vi "HDI Fiducial.vi"(5 "error in (no error)":errorcluster, 6 "Image Src":T1) -> (0 "Matched?":bool, 1 "y rel move":dbl, 2 "x rel move":dbl, 3 "Score":dbl, 4 "error out":errorcluster)   [LabVIEW 2011]
uses:
  <vilib>/vision/Pattern Matching.llb/IMAQ GM Match Report.ctl
  <vilib>/vision/Image Controls.llb/IMAQ Image.ctl
  <vilib>/vision/Pattern Matching.llb/IMAQ Curve Parameters.ctl
  <vilib>/vision/Pattern Matching.llb/IMAQ Match Range Setting.ctl
  <vilib>/vision/NI_Vision_Development_Module.lvlib
panel:
  in  "Scale Factor":sgl=0.000429
  out "y":sgl
  out "x":sgl
  out "Image Out":T1(plugin-control)
  out "Calibrated Matches (Geometric Matching 1)":T2[](array[typedef]) {"Correlation Score" format="%.2f"; "Target Template Curve Score" format="%.2f"; "Template Target Curve Score" format="%.2f"; "Bounding Box"."y" format="%.2f"; "Bounding Box"."x" format="%.2f"; "Position"."y" format="%.2f"; "Position"."x" format="%.2f"; "Score" format="%.2f"; "Scale" format="%.2f"; "Angle" format="%.2f"; "Occlusion %" format="%.2f"}
  out "Matches (Geometric Matching 1)":T2[](array[typedef]) {"Correlation Score" format="%.2f"; "Target Template Curve Score" format="%.2f"; "Template Target Curve Score" format="%.2f"; "Bounding Box"."y" format="%.2f"; "Bounding Box"."x" format="%.2f"; "Position"."y" format="%.2f"; "Position"."x" format="%.2f"; "Score" format="%.2f"; "Scale" format="%.2f"; "Angle" format="%.2f"; "Occlusion %" format="%.2f"}
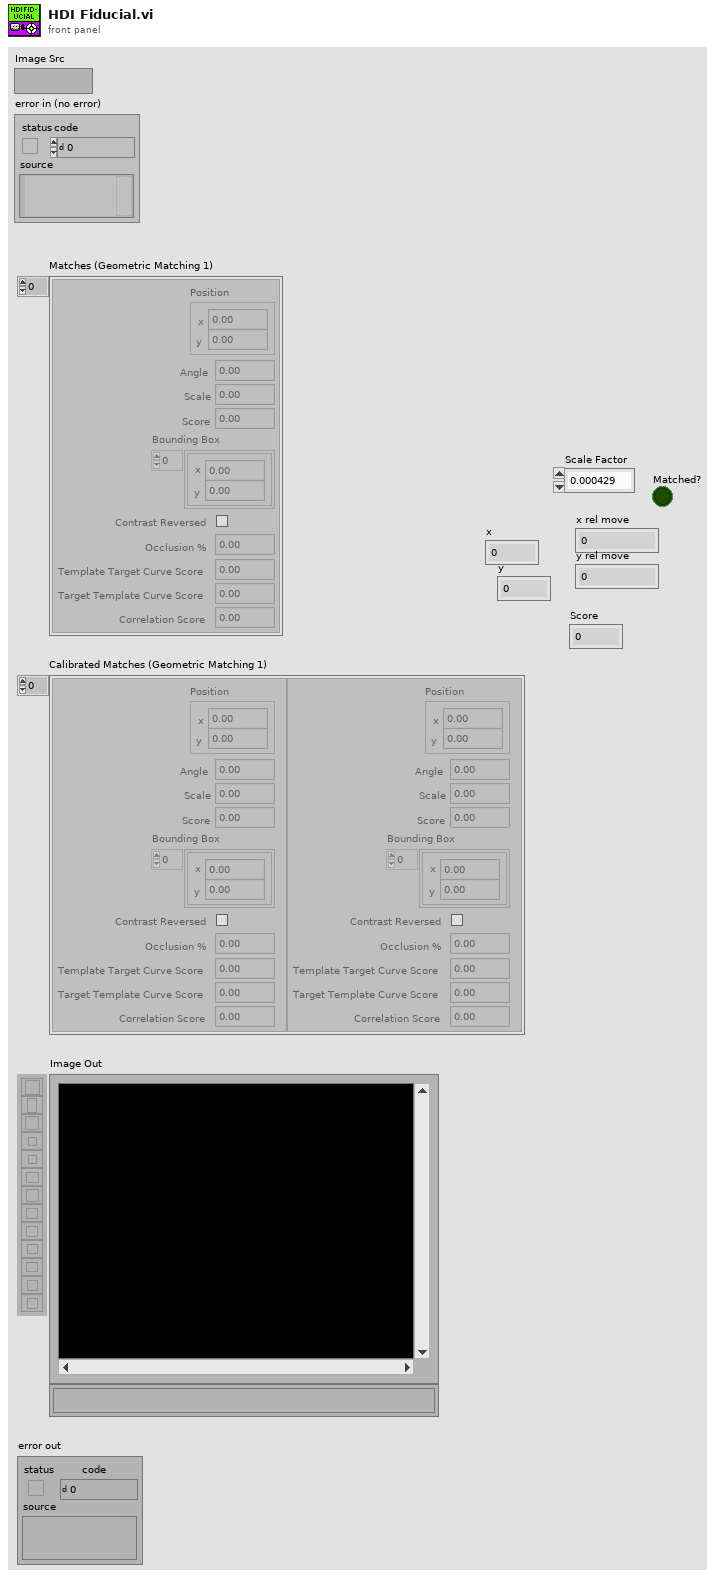
[diagram p1: front panel]
types:
  T1 = typedef "IMAQ Image.ctl" = refnum<image>
  T2 = typedef "IMAQ GM Match Report.ctl" = cluster{"Position":cluster{"x":sgl, "y":sgl}, "Angle":sgl, "Scale":sgl, "Score":sgl, "Bounding Box":cluster{"x":sgl, "y":sgl}[], "Contrast Reversed":bool, "Occlusion %":sgl, "Template Target Curve Score":sgl, "Target Template Curve Score":sgl, "Correlation Score":sgl}
  T3 = typedef "IMAQ Curve Parameters.ctl" = cluster{"Extraction Mode":u32, "Edge Threshold":i32, "Edge Filter Size":u32, "Min Length":i32, "Row Search Step Size":i32, "Col Search Step Size":i32, "Max Endpoint Gap":i32, "Closed":bool, "Subpixel":bool}
  T4 = typedef "IMAQ Match Range Setting.ctl" = cluster{"Match Constraints":u32, "Min":dbl, "Max":dbl}
  T5 = cluster{"Curve Parameters":T3, "Match Mode":cluster{"Rotation":bool, "Scale":bool, "Occlusion":bool, "Reserved":bool, "Reserved":bool, "Reserved":bool}, "Range Settings":T4[], "Number of Matches":i32, "Minimum Match Score":sgl, "SubPixel Accuracy":bool, "Adv. Geometric Match Options 2":cluster{"Setup Data Item":u16, "Item Value":dbl}[]}
  T6 = cluster{"Global Rectangle":i32[], "Contours":cluster{"ID":enum32{"External", "Internal"}, "Type":u32, "Coordinates":i32[]}[]}
  T7 = cluster{"histogram":u32[], "Minimal Value":sgl, "Maximal Value":sgl, "Starting Value":sgl, "Interval Width":sgl, "Mean Value":sgl, "Standard  Variation":sgl, "Area (pixels)":i32}
  T8 = typedef "Image Type" = u32
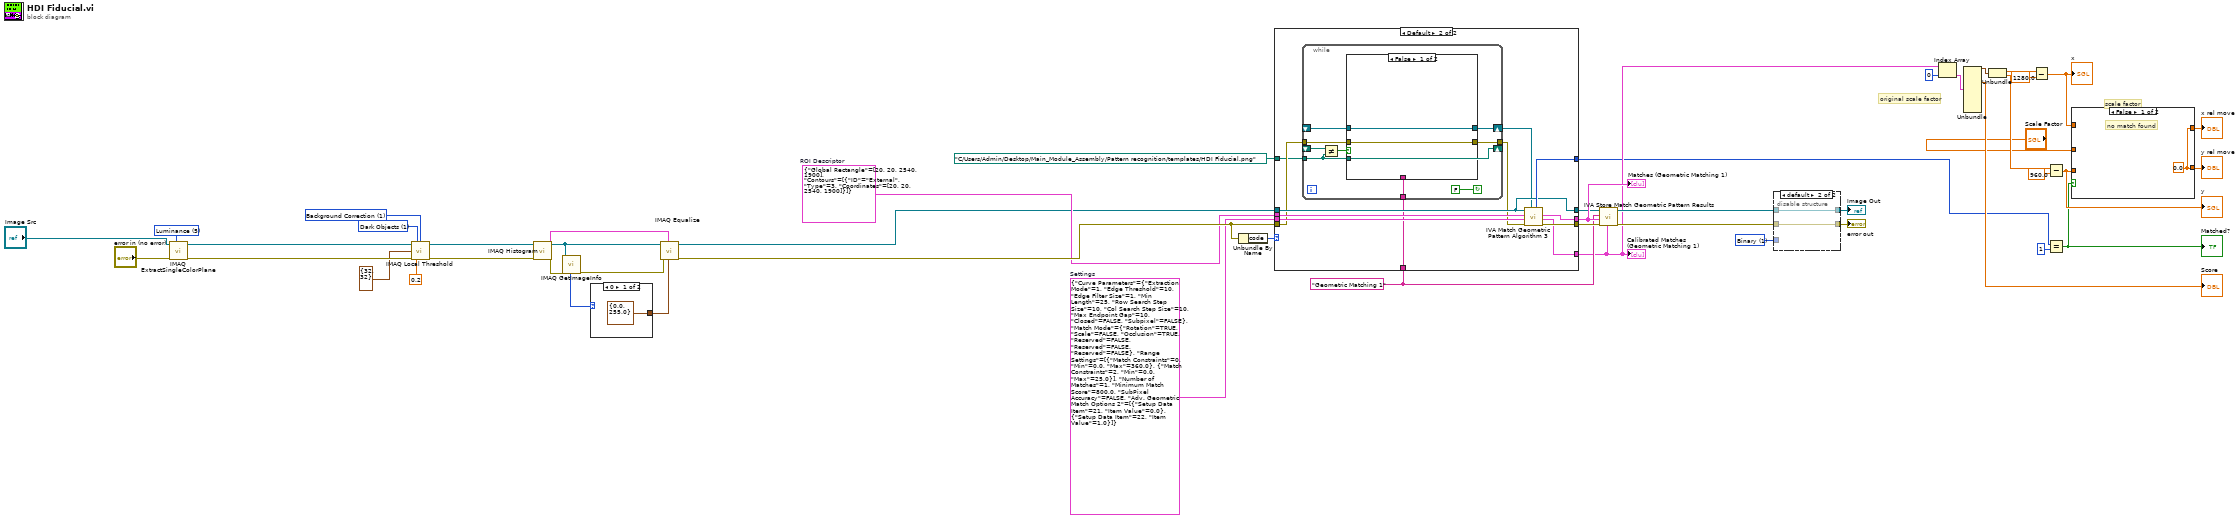
[diagram p0: block diagram]
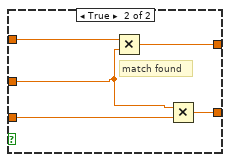
[diagram p2: hidden frame]
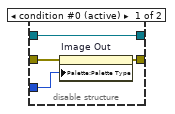
[diagram p3: hidden frame]
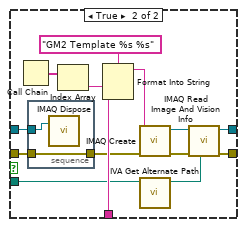
[diagram p5: hidden frame]
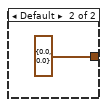
[diagram p6: hidden frame]
diagram:
  w20 = u32 1 items=["Grayscale", "Binary", "Gradient", "Rainbow", "Temperature", "User Defined"] ("Palette")
  w25 = T5 {"Curve Parameters"={"Extraction Mode"=1, "Edge Threshold"=10, "Edge Filter Size"=1, "Min Length"=25, "Row Search Step Size"=10, "Col Search Step Size"=10, "Max Endpoint Gap"=10, "Closed"=FALSE, "Subpixel"=FALSE}, "Match Mode"={"Rotation"=TRUE, "Scale"=FALSE, "Occlusion"=TRUE, "Reserved"=FALSE, "Reserved"=FALSE, "Reserved"=FALSE}, "Range Settings"=[{"Match Constraints"=0, "Min"=0.0, "Max"=360.0}, {"Match Constraints"=2, "Min"=0.0, "Max"=25.0}], "Number of Matches"=1, "Minimum Match Score"=800.0, "SubPixel Accuracy"=FALSE, "Adv. Geometric Match Options 2"=[{"Setup Data Item"=21, "Item Value"=0.0}, {"Setup Data Item"=22, "Item Value"=1.0}]}  # Settings
  w24 = "Geometric Matching 1" ("Step Name")
  w32 = T6 {"Global Rectangle"=[20, 20, 2540, 1900], "Contours"=[{"ID"=enum."External", "Type"=3, "Coordinates"=[20, 20, 2540, 1900]}]}  # ROI Descriptor
  w42 = u32 1 items=["Bright Objects", "Dark Objects"] ("Look For (Bright Objects)")
  w45 = u32 1 items=["Niblack", "Background Correction"] ("Method")
  w48 = 5 items=["Red", "Green", "Blue", "Hue", "Saturation", "Luminance", "Value", "Intensity"] ("Color Plane")
  # "original scale factor"
  # "scale factor"
  n1 = call "IMAQ ExtractSingleColorPlane"("Color Plane"=w48, "error in (no error)"="error in (no error)", "Image Src"="Image Src") -> ("error out"=w47:errorcluster, "Image Dst Out"=w46:T1)  [unwired: 1 in, 6 out]
  n2 = call "IMAQ Local Threshold"("Image Src"=w46, "Look For (Bright Objects)"=w42, "Method (Niblack)"=w45, "Window Size (32x32)"=cluster{"SizeX":i32, "SizeY":i32} {"SizeX"=32, "SizeY"=32} ("Kernel Size"), "error in (no error)"=w47, "Niblack Deviation Factor (0.2)"=0.2 ("Niblack Deviation Factor")) -> ("Image Dst Out"=w37:T1, "error out"=w41:errorcluster)  [unwired: 2 in, 6 out]
  n3 = call "IMAQ Histogram"("error in (no error)"=w41, "Image"=w37) -> ("error out"=w36:errorcluster, "Histogram Report"=w39:T7)  [unwired: 3 in, 5 out]
  n4 = call "IMAQ GetImageInfo"("error in (no error)"=w36, "Image"=w37) -> ("error out"=w35:errorcluster, "Image Type"=w38:T8)  [unwired: 8 out]
  n5 = case shown="0" w38 {
    tunnel: [cluster{"Minimum":sgl, "Maximum":sgl} {"Minimum"=0.0, "Maximum"=255.0} ("Range") cluster{"Minimum":sgl, "Maximum":sgl} {"Minimum"=0.0, "Maximum"=0.0} ("Range")] -> w34
    frame 0 {
    }
    frame Default {
    }
  }
  n6 = call "IMAQ Equalize"("Range"=w34, "Histogram Report"=w39, "error in (no error)"=w35, "Image Src"=w37) -> ("error out"=w40:errorcluster, "Image Dst Out"=w31:T1)  [unwired: 2 in, 4 out]
  n7 = Unbundle By Name(w40) -> ("code"=w27:i32)
  n8 = case shown="Default" w27 {
    tunnel: path "C:/Users/Admin/Desktop/Main_Module_Assembly/Pattern recognition/templates/HDI Fiducial.png" ("Template File Path") -> [_ w53]
    tunnel: w40 -> [_ w54]
    tunnel: w25 -> [_ w63]
    tunnel: w32 -> [_ w62]
    tunnel: w31 -> [w51 w57]
    tunnel: [_ w61] -> w30
    tunnel: [_ w60] -> w28
    tunnel: [_ w59] -> w4
    tunnel: [_ w58] -> w3
    tunnel: [w51 w57] -> w26
    tunnel: w24 -> [_ w52]
    frame -1074396199, -1074396198 {
      # "Discard Coordinate System Error"
    }
    frame Default {
      n9 = while {
        shift-right: [w72] -> w55
        shift-left: _ -> [w71]
        tunnel: [w69] -> w56
        tunnel: w54 -> [w68]
        tunnel: w53 -> [w64]
        tunnel: w52 -> [w67]
        shift-right: [w64] -> _
        shift-left: _ -> [w66]
        stop <- FALSE continue-if-true
        n10 = Not Equal?(x=w66, y=w64) -> (x != y?=w65:bool)
        n11 = case shown="False" w65 {
          tunnel: [w74 w86] -> w72
          tunnel: w71 -> [w74 w78]
          tunnel: [w73 w83] -> w69
          tunnel: w68 -> [w73 w79]
          tunnel: w67 -> [_ w80]
          tunnel: w64 -> [_ w76]
          frame False {
          }
          frame True {
            n12 = Call Chain() -> (call chain=w82:string[])
            n13 = stacked-sequence {
              tunnel: w79 -> [w90]
              tunnel: w78 -> [w89]
              tunnel: [w90] -> w77
              frame #0 {
                n14 = call "IMAQ Dispose"("Image"=w89) -> ()  [unwired: 2 in, 4 out]
              }
            }
            n15 = Index Array(array=w82) -> (element=w81:string)  [unwired: 1 in]
            n16 = Format Into String(format string="GM2 Template %s %s" ("Image Name"), w81, w80) -> (resulting string=w88:string)  [unwired: 2 in, 1 out]
            n17 = call "IMAQ Create"("Image Name"=w88, "error in (no error)"=w77) -> ("New Image"=w85:T1, "error out"=w84:errorcluster)  [unwired: 2 in, 1 out]
            n18 = call <vilib>:"IVA Get Alternate Path.vi"("Path In"=w76) -> ("Path Out"=w75:path)  [unwired: 10 out]
            n19 = call "IMAQ Read Image And Vision Info"("File Path"=w75, "error in (no error)"=w84, "Image"=w85) -> ("error out"=w83:errorcluster, "Image Out"=w86:T1)  [unwired: 1 in, 6 out]
          }
        }
      }
      n20 = call <vilib>:"IVA Match Geometric Pattern Algorithm 3.vi"("Template"=w55, "error in (no error)"=w56, "Settings"=w63, "ROI Descriptor"=w62, "Image"=w57) -> ("error out"=w61:errorcluster, "Calibrated Matches"=w59:T2[], "Matches"=w60:T2[], "Number of Matches"=w58:i32)  [unwired: 3 out]
    }
  }
  "Matches (Geometric Matching 1)" <- w28
  "Calibrated Matches (Geometric Matching 1)" <- w4
  n21 = call <vilib>:"IVA Store Match Geometric Pattern Results.vi"("Calibrated Matches"=w4, "error in (no error)"=w30, "Matches"=w28, "Step Name"=w24, "Image in"=w26) -> ("error out"=w29:errorcluster, "Image dup"=w22:T1)  [unwired: 5 out]
  n22 = disable-structure "Conditional Disable Structure" shown="default" {
    disable-tunnel: w29 -> [w94 w95]
    disable-tunnel: [w93 w95] -> w23
    disable-tunnel: w22 -> [w92 w96]
    disable-tunnel: [w92 w96] -> w21
    disable-tunnel: w20 -> [w91 _]
    frame condition #0 (active) {
      n23 = property on="Image Out" class="ImageControl"(error in=w94, "Palette:Palette Type"=w91) -> (error out=w93:errorcluster)  [unwired: 1 in, 1 out]
    }
    frame condition #1 {
    }
  }
  "error out" <- w23
  "Image Out" <- w21
  n24 = Index Array(array=w4, index=0) -> (element=w10:T2)
  n25 = Unbundle(w10) -> ("Position"=w7:cluster{"x":sgl, "y":sgl}, "Score"=→"Score":sgl)  [unwired: 8 out]
  n26 = Unbundle(w7) -> ("x"=w9:sgl, "y"=w8:sgl)
  n27 = Subtract(x=w9, y=sgl 1280.0) -> (x-y=w16:sgl)
  "x" <- w16
  n28 = Subtract(x=w8, y=sgl 960.0) -> (x-y=w17:sgl)
  "y" <- w17
  n29 = Equal?(x=w3, y=1) -> (x = y?=w14:bool)
  "Matched?" <- w14
  n30 = case shown="False" w14 {
    tunnel: w17 -> [_ w102]
    tunnel: w16 -> [_ w101]
    tunnel: [w97 w100] -> w13
    tunnel: [w97 w99] -> w12
    tunnel: "Scale Factor" -> [_ w98]
    frame False {
      w97 = sgl 0.0
      # "no match found"
    }
    frame True {
      # "match found"
      n31 = Multiply(x=w101, y=w98) -> (x*y=w100:sgl)
      n32 = Multiply(x=w98, y=w102) -> (x*y=w99:sgl)
    }
  }
  "x rel move" <- w13
  "y rel move" <- w12
